vi "countrate.vi"() -> ()   [LabVIEW 2015]
uses:
  <vilib>/platform/TimedLoop/XDataNode/XDataNode.xnode
  <vilib>/Platform/TimedLoop/XDataNode/nitl_modes.ctl
  <vilib>/Platform/TimedLoop/XDataNode/XDNodeRunTimeDep.lvlib
  <vilib>/Platform/TimedLoop/XDataNode/wakeup.ctl
  <vilib>/Platform/TimedLoop/XDataNode/timing_clust.ctl
  <vilib>/Utility/file.llb/Write Delimited Spreadsheet (I64).vi
panel:
  out "Waveform Graph":i32[](graph)
  in  "Total Time (s)":dbl
  in  "Time Increment (s)":dbl
  out "counts per second":dbl(knob) scale=0.0..100.0
  in  "stop":bool
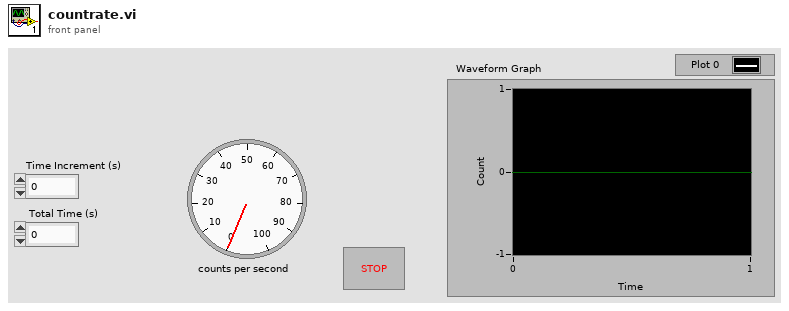
[diagram p1: front panel]
types:
  T1 = typedef "XDNodeRunTimeDep.lvlib/timing_clust.ctl" = cluster{"Expected End [f-1]":u64, "Actual End [f-1]":u64, "Finished Late? [f-1]":bool, "Expected End [i-1]":u64, "Actual End [i-1]":u64, "Finished Late? [i-1]":bool, "Expected Start [i]":u64, "Actual Start [i]":u64, "Expected Start [f]":u64, "Actual Start [f]":u64, "Source Name":string, "Structure Name":string, "Period":i64, "Deadline":i64, "Offset":i64, "Start":i64, "Priority":i32, "Timeout":i32, "Mode":T2, "Wakeup Reason":T3, "Error":errorcluster, "Source Type":string, "Secondary Source Type":string, "Global End Time":u64, "Global Start Time":u64, "Frame Duration":u64, "Iteration Duration":u64, "Assigned CPU":i32, "I/O Scan Engine Mode":u32}
  T2 = typedef "XDNodeRunTimeDep.lvlib/nitl_modes.ctl" = enum32{"No Change", "Process missed periods, maintain original phase", "Discard missed periods, maintain original phase", "Process missed periods, ignore original phase", "Discard missed periods, ignore original phase"}
  T3 = typedef "XDNodeRunTimeDep.lvlib/wakeup.ctl" = enum32{"Normal", "Aborted", "Asynchronous wakeup", "Timing source error", "Timed loop error", "Timeout"}
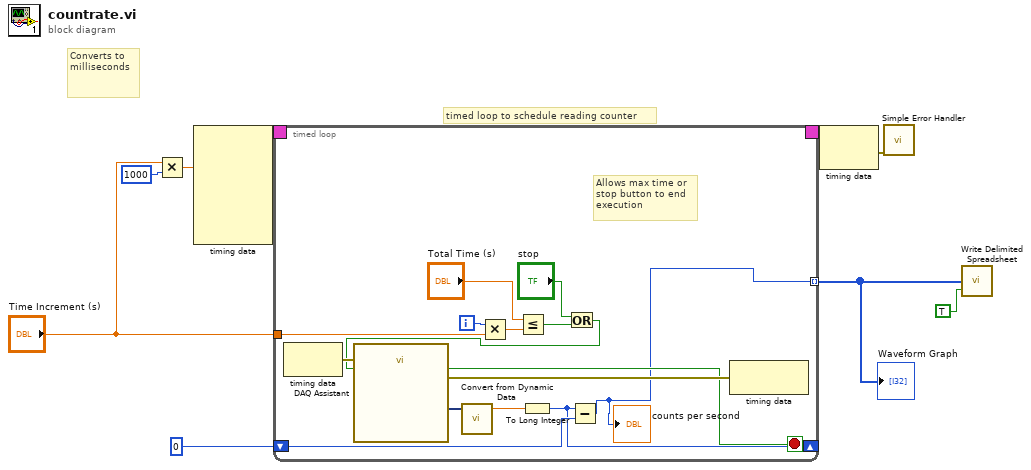
[diagram p0: block diagram]
diagram:
  # "Converts to milliseconds"
  # "timed loop to schedule reading counter"
  n1 = Multiply(x="Time Increment (s)", y=1000) -> (x*y=w3:dbl)
  n2 = node-c288(w3) -> (w9:T1)  [unwired: 5 in]
  n3 = timed-loop {
    timing: w9 -> [_]
    timing-out: [_] -> w8
    shift-right: [w22] -> _
    shift-left: 0 -> [w23]
    tunnel: "Time Increment (s)" -> [w18]
    tunnel: [w10] -> w1 mode=indexing
    i -> [w17]
    stop <- w11 stop-if-true
    # "Allows max time or stop button to end execution"
    n4 = node-c288() -> (w19:errorcluster)  [unwired: 1 in]
    n5 = Multiply(x=w17, y=w18) -> (x*y=w15:dbl)
    n6 = Less Or Equal?(x="Total Time (s)", y=w15) -> (x <= y?=w14:bool)
    n7 = Or(x="stop", y=w14) -> (x .or. y?=w12:bool)
    n8 = call "DAQ Assistant"("error in"=w19, "stop (F)"=w12) -> ("data"=w24:dynamicdata, "stopped"=w11:bool, "error out"=w20:errorcluster)  [unwired: 14 in, 1 out]
    n9 = call "Convert from Dynamic Data"("Dynamic Data Type"=w24) -> ("Scalar"=w21:dbl)  [unwired: 3 in]
    n10 = To Long Integer(number=w21) -> (32bit integer=w22:i32)
    n11 = Subtract(x=w22, y=w23) -> (x-y=w10:i32)
    "counts per second" <- w10
    n12 = node-c288(w20) -> ()  [unwired: 1 out]
  }
  "Waveform Graph" <- w1
  n13 = node-c288(w8) -> (w6:errorcluster)
  n14 = call <vilib>:"Simple Error Handler.vi"("error in (no error)"=w6) -> ()  [unwired: 4 in, 5 out]
  n15 = call-poly <vilib>:"Write Delimited Spreadsheet.vi"("1D data"=w1, "transpose? (F)"=TRUE) -> ()  [unwired: 12 in, 2 out]
